vi "Scale Demo.vi"() -> (1 "picture":picture)   [LabVIEW 2010]
doc: "Uses the Calc Scale Specs VI and the Draw Scale VI to draw a scale of a Cartesian graph in a picture indicator. You can change the range, location, and orientation of the scale. The Polar Graph VIs and the Cartesian Graph VIs also use the Scale VIs to draw the scales for the graphs.\n\nNote: You must have the LabVIEW Full or Professional Development Systems to run this example."
panel:
  in  "tick mark length":i16=11
  in  "constant coordinate":i16=19
  in  "scale definition":T1={"coordinate 1"=9, "value 1"=5.0, "coordinate 2"=55, "value 2"=10.0, "log"=FALSE, "fmt and prec"={"format"=enum."Hex", "precision"=2}} {"value 2" format="%0.2f"; "value 1" format="%0.2f"}
  in  "scale attributes":T2={"horizontal"=TRUE, "left/top"=FALSE, "draw bar"=TRUE, "line color"=255, "text color"=0}
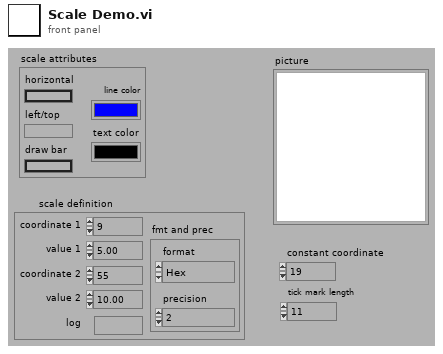
[diagram p1: front panel]
types:
  T1 = cluster{"coordinate 1":i16, "value 1":dbl, "coordinate 2":i16, "value 2":dbl, "log":bool, "fmt and prec":cluster{"format":enum8{"Decimal", "Scientific", "Engineering", "Binary", "Octal", "Hex"}, "precision":u8}}
  T2 = cluster{"horizontal":bool, "left/top":bool, "draw bar":bool, "line color":u32, "text color":u32}
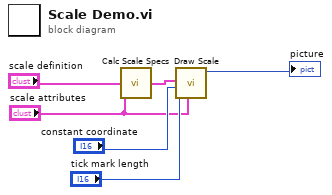
[diagram p0: block diagram]
diagram:
  n1 = call <vilib>:"Calc Scale Specs.vi"("scale definition"="scale definition", "scale attributes"="scale attributes") -> ("scale specs"=w5:cluster{"coordinate":i16, "label":string}[])  [unwired: 2 in, 5 out]
  n2 = call <vilib>:"Draw Scale.vi"("scale attributes"="scale attributes", "tick length(3)"="tick mark length", "constant coordinate"="constant coordinate", "scale specs"=w5) -> ("new picture"=→"picture":picture)  [unwired: 3 in, 4 out]
